vi "Determine Warnings 3-5.vi"() -> ()   [LabVIEW 2014]
panel:
  out "Warning?":bool
  out "Warning Text":string
  in  "Min Temp":dbl
  in  "Max Temp":dbl
  in  "Current Temp":dbl
  # "If you have a min temp that is greater than your max temp then the warning text will be \ndetermined by the the Current Temps value"
  # "18."
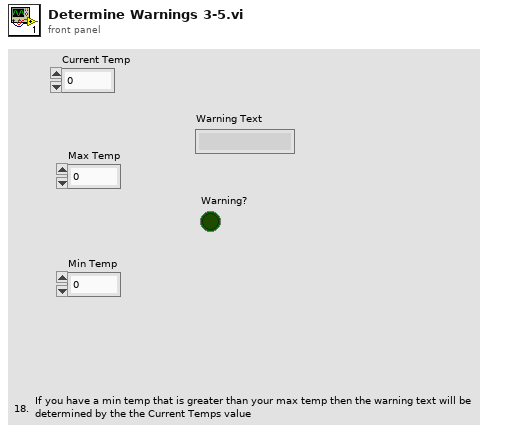
[diagram p1: front panel]
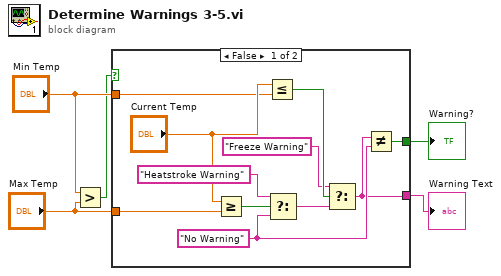
[diagram p0: block diagram]
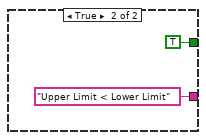
[diagram p2: hidden frame]
diagram:
  n1 = Greater?(x="Min Temp", y="Max Temp") -> (0:w1:bool)
  n2 = case shown="False" w1 {
    tunnel: [w12 TRUE] -> w5
    tunnel: [w8 "Upper Limit < Lower Limit"] -> w4
    tunnel: "Min Temp" -> [w7 _]
    tunnel: "Max Temp" -> [w6 _]
    frame False {
      w13 = "No Warning"
      n3 = Greater Or Equal?(x="Current Temp", y=w6) -> (x >= y?=w15:bool)
      n4 = Less Or Equal?(x="Current Temp", y=w7) -> (x <= y?=w14:bool)
      n5 = Select(t="Heatstroke Warning", s=w15, f=w13) -> (s? t:f=w10:string)
      n6 = Select(t="Freeze Warning", s=w14, f=w10) -> (s? t:f=w8:string)
      n7 = Not Equal?(x=w8, y=w13) -> (x != y?=w12:bool)
    }
    frame True {
    }
  }
  "Warning Text" <- w4
  "Warning?" <- w5
